vi "Enqueue Message_TICO behavior.vi"   [LabVIEW 2025]
doc: "For a regular message, enqueue the message. For a priority message, enqueue it at the front of the queue."
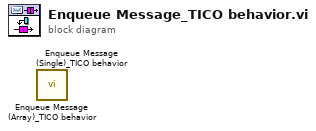
[diagram p0: block diagram]
diagram:
  n1 = call "Enqueue Message (Array)_TICO behavior.vi"() -> ()  [unwired: 10 in, 2 out]
  n2 = call "Enqueue Message (Single)_TICO behavior.vi"() -> ()  [unwired: 10 in, 2 out]
